vi "Open_File_for_Read.vi"(11 "file path":path) -> (0 "error out":errorcluster, 1 "exists?":bool, 2 "Permission error?":bool, 3 "refnum":refnum<file>)   [LabVIEW 2010]
doc: "Opens an existing file, creates a new file, or replaces an existing file, programmatically or interactively using dialog. You can optionally specify a dialog prompt, default file name, start path, or filter pattern, and you can specify open and deny modes when opening a file, plus group and permission when creating a new file. Use this VI with the intermediate Write File+ or Read File+ VIs described below.\n\nfile path is the path name of the file. If file path is empty (default value) or is Not A Path, the VI displays a File dialog box from which you can select a file. Error 43 occurs if the user cancels the dialog. \n\nfunction is the operation to perform:\n\n 0 (open) opens an existing file. Error 7 occurs if the file cannot be found.\n \n 1 (open or create) opens an existing file or creates a new file if one does not exist.\n\n 2 (create or replace) creates a new file or replaces a file if it exists and you give permission. Replacement is done by opening the file and setting EOF to 0. Error 43 occurs if the user elects to disallow the replacement using dialog. \n\n 3 (create) creates a new file. Error 8 occurs if the file already exists.\n\nadvisory dialog? Set TRUE (default) if you want a dialog if function=0 and the file does not exist, or if function=2 or 3 and the file exists.\n\nprompt is the message that appears below the list of files and directories in the file dialog.\n\ndefault name is the initial file name that appears in the selection box of the file dialog.\n\nstart path is the path name to the initially displayed directory in a file dialog. The default value is Not A Path, which is the path to the last directory shown in a file dialog.\n\npattern is the match pattern specification to display only certain types of files or directories. See the description of the File Dialog function for more information.\n\nerror in is a cluster of three elements (error?, code, and source) that describe the upstream error state, that is, the existance of any error preceeding the execution of the VI. The VI executes normally only if no incoming error exists; otherwise it merely passes the error in value to error out. error? is TRUE if an error occurred; the default value is FALSE. code is the error code; the default value is 0. source is in most cases the name of the VI or function that produced the error; the default value is an empty string.\n\nnew file path is the path of the file opened or created. You can use this output to determine the path of a file that you open or create using dialog. new file path returns Not A Path if the user selects Cancel from the dialog box.\n\nrefnum is the reference number of the open file. The value is Not A Refnum if the file cannot be opened.\n\nfile size is the size of the file in bytes; it is also the location of the end of file.\n\nerror out is a cluster of three elements (error?, code, and source) that describe the error state following the execution of the VI. If an incoming error does not exist, the VI executes normally and error out describes the VI's error state; if an incoming error exists, error out equals error in."
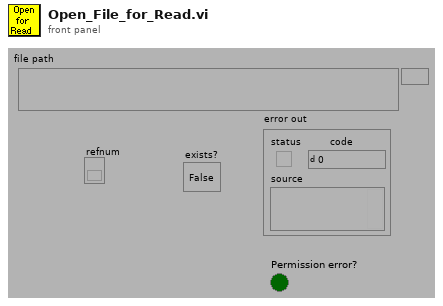
[diagram p1: front panel]
types:
  T1 = enum16{"read/write", "read-only", "write-only", "write-only (truncate)"}
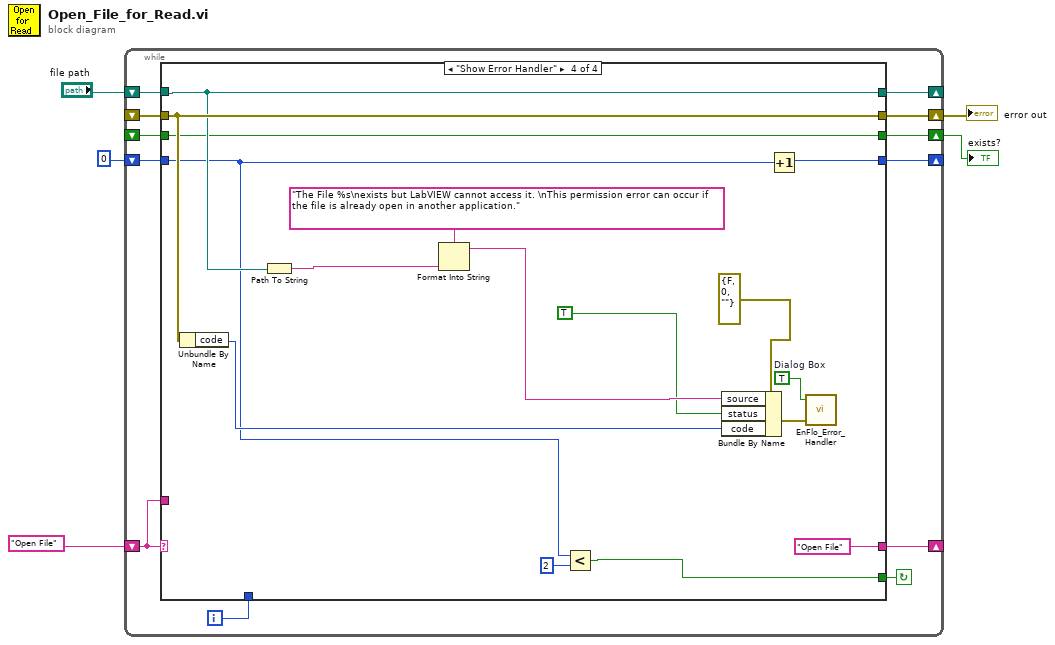
[diagram p0: block diagram]
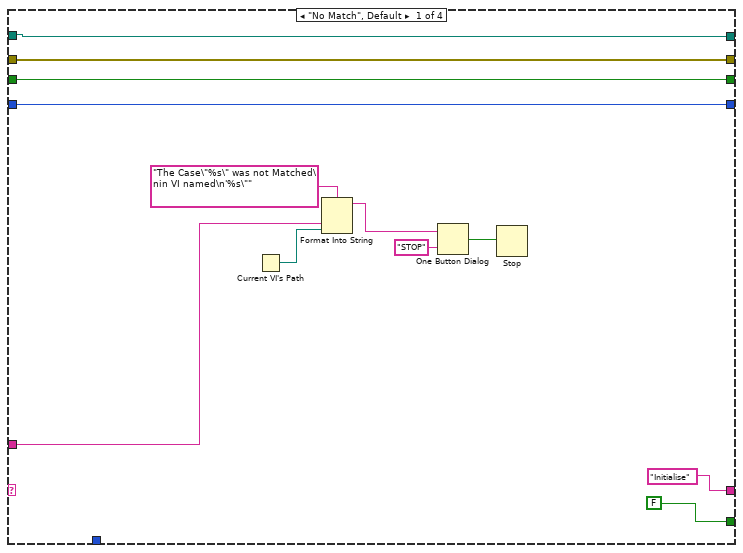
[diagram p2: hidden frame]
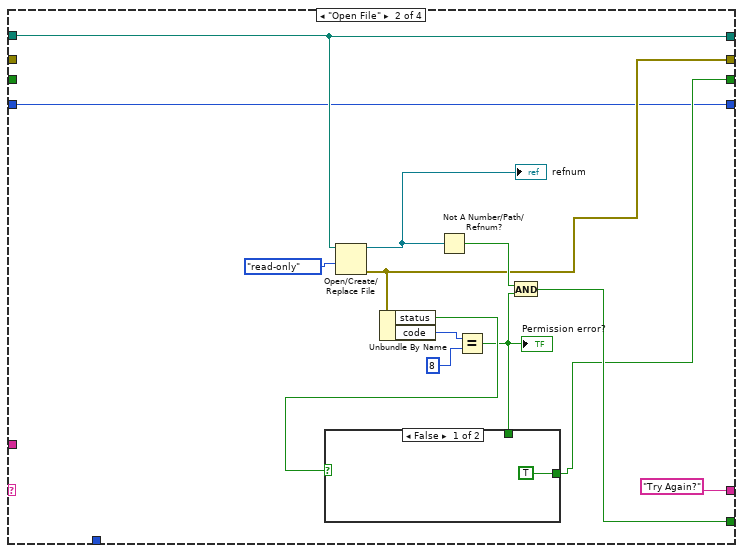
[diagram p3: hidden frame]
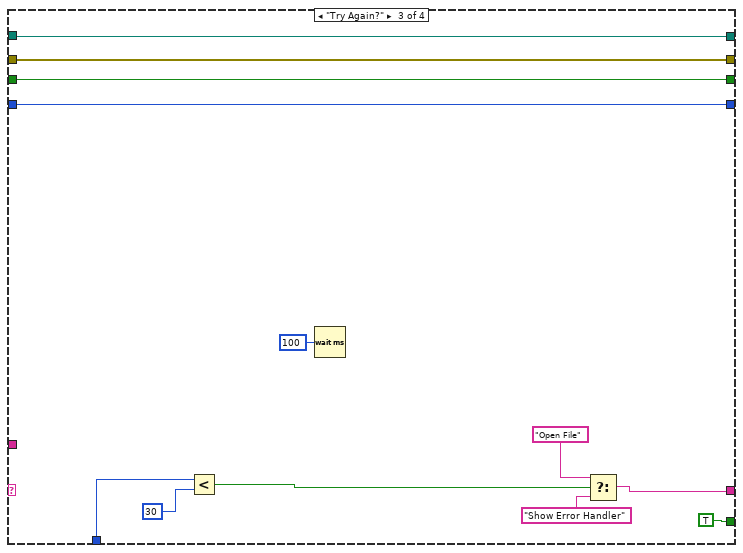
[diagram p5: hidden frame]
diagram:
  n1 = while {
    shift-left: "Open File" -> [w15]
    shift-right: [w16] -> _
    shift-right: [w13] -> w4
    shift-left: _ -> [w10]
    shift-right: [w11] -> _
    shift-left: "file path" -> [w12]
    shift-right: [w8] -> w2
    shift-left: _ -> [w9]
    shift-right: [w6] -> _
    shift-left: 0 -> [w7]
    i -> [w14]
    stop <- w17 continue-if-true
    n2 = case shown="\"Show Error Handler\"" w15 {
      tunnel: [FALSE w35 TRUE w59] -> w17
      tunnel: ["Initialise" "Try Again?" w51 "Open File"] -> w16
      tunnel: w15 -> [w24 _ _ _]
      tunnel: w12 -> [w21 w40 w47 w71]
      tunnel: w14 -> [_ _ w54 _]
      tunnel: [w20 w34 w48 w72] -> w13
      tunnel: [w21 w40 w47 w71] -> w11
      tunnel: w10 -> [w20 _ w48 w72]
      tunnel: w9 -> [w19 _ w46 w62]
      tunnel: [w19 w31 w46 w62] -> w8
      tunnel: w7 -> [w18 w30 w45 w58]
      tunnel: [w18 w30 w45 w57] -> w6
      frame "No Match", Default {
        n3 = Current VI's Path() -> (path=w23:path)
        n4 = Format Into String(format string="The Case\"%s\" was not Matched\nin VI named\n'%s\"" ("Format String"), w24, w23) -> (resulting string=w27:string)  [unwired: 2 in, 1 out]
        n5 = One Button Dialog(message=w27, button name ("OK")="STOP") -> (true=w25:bool)
        n6 = Stop(stop? (T)=w25) -> ()
      }
      frame "Open File" {
        n7 = Open/Create/Replace File(file path (use dialog)=w40, access (0:read/write)=T1."read-only" ("open mode (0)")) -> (refnum out=w39:refnum<file>, error out=w34:errorcluster)  [unwired: 1 in, 4 out]
        "refnum" <- w39
        n8 = Unbundle By Name(w34) -> ("status"=w33:bool, "code"=w38:i32)
        n9 = Not A Number/Path/Refnum?(number/path/refnum=w39) -> (NaN/Path/Refnum?=w36:bool)
        n10 = Equal?(x=w38, y=8) -> (x = y?=w32:bool)
        "Permission error?" <- w32
        n11 = case shown="False" w33 {
          tunnel: [TRUE w44] -> w31
          tunnel: w32 -> [_ w44]
          frame False {
          }
          frame True {
          }
        }
        n12 = And(x=w36, y=w32) -> (x .and. y?=w35:bool)
      }
      frame "Try Again?" {
        n13 = Less?(x=w54, y=30) -> (x < y?=w52:bool)
        n14 = Wait (ms)(milliseconds to wait=u32 100) -> ()  [unwired: 1 out]
        n15 = Select(t="Open File", s=w52, f="Show Error Handler") -> (s? t:f=w51:string)
      }
      frame "Show Error Handler" {
        w70 = TRUE  # Dialog Box
        n16 = Unbundle By Name(w72) -> ("code"=w66:i32)
        n17 = Path To String(path=w71) -> (string=w63:string)
        n18 = Format Into String(format string="The File %s\nexists but LabVIEW cannot access it. \nThis permission error can occur if the file is already open in another application." ("Format String"), w63) -> (resulting string=w67:string)  [unwired: 2 in, 1 out]
        n19 = Less?(x=w58, y=2) -> (x < y?=w59:bool)
        n20 = Bundle By Name(cluster=errorcluster {"status"=FALSE, "code"=0, "source"=""} ("error in (no error)"), "source"=w67, "status"=TRUE, "code"=w66) -> (w69:errorcluster)
        n21 = Increment(x=w58) -> (x+1=w57:i32)
        n22 = call "EnFlo_Error_Handler.vi"("error in (no error)"=w69, "Dialog Box (T)"=w70) -> ()  [unwired: 1 in, 3 out]
      }
    }
  }
  "error out" <- w4
  "exists?" <- w2
